vi "2014 Target Detection.vi"() -> (2 "Target Info":T4(array[cluster]))   [LabVIEW 2013]
uses:
  TargetType.ctl
  <vilib>/Rock Robotics/WPI/Camera/WPI_CameraImageSize.ctl
  <vilib>/Rock Robotics/WPI/Camera/WPI_CameraWhite Balance Values.ctl
  <vilib>/Rock Robotics/WPI/Camera/WPI_CameraExposure Values.ctl
  <vilib>/Rock Robotics/WPI/Camera/WPI_CameraFrameRate.ctl
panel:
  in  "Range":cluster{"Lower value":sgl, "Upper value":sgl}={"Lower value"=150.0, "Upper value"=255.0} {"Lower value" scale=0.0..255.0; "Upper value" scale=0.0..255.0}
  in  "Image Size":T1=enum."320x240"
  in  "error in (no error)":errorcluster
  in  "Instructions:":string="Images:\nUse the tab immediately below to choose the image source. Update the camera settings or the image directory so that you have images or video to test with.\n\nCalibration:\nYou can update Color Component ranges directly, or by clicking and drawing a line on the colored strip in the Image control. The Std Dev multipliers and where the strip is drawn determine the calibration values.\n\nUse Debugging tab to view the result of the color range threshold .\n\nArea Size LImit is used to ignore objects too small or far away to care about.\n\nThe Details tab contains score details for each target and subObject.\n\nCamera Type is used to select lens angles for distance calculation.\n\nVertical strips with no adjacent horizontal strip are identified as \"not hot\" and marked in blue.\nThe numeric scores indicate represent aspect ratio and rectangularity.\n\nWhen both strips are near enough, the pair is identified as \"hot\" and marked in green. Scores\nindicate the left, right, ratio of widths, and vertical positioning.\n\nAny score that falls below cutoff is drawn in red and bounding box is drawn in red."
  in  "Std Devs":cluster{"Hue":dbl, "Sat":dbl, "Val":dbl}={"Hue"=4.0, "Sat"=6.0, "Val"=4.0}
  in  "Area Size Limit %":dbl=0.06 format="%#_13g"
  in  "Camera Type":enum16{"206", "1011", "1013"}(ring)=enum."1013"
  out "loop time ms":u32
  in  "Score Cutoff":dbl(slide)=54.248366013071895 scale=0.0..100.0
  in  "Image Source":enum32{"Files", "Camera"}(tab)
  in  "List of image files":i32(listbox)
  in  "Image Directory":path=path "2014 Pseudo-Target/2014 Pseudo-Target Active"
  in  "Tabbed Info":enum32{"Debugging", "Details"}(tab)
  out "Mask":T2(plugin-control)
  out "Image":T2(plugin-control)
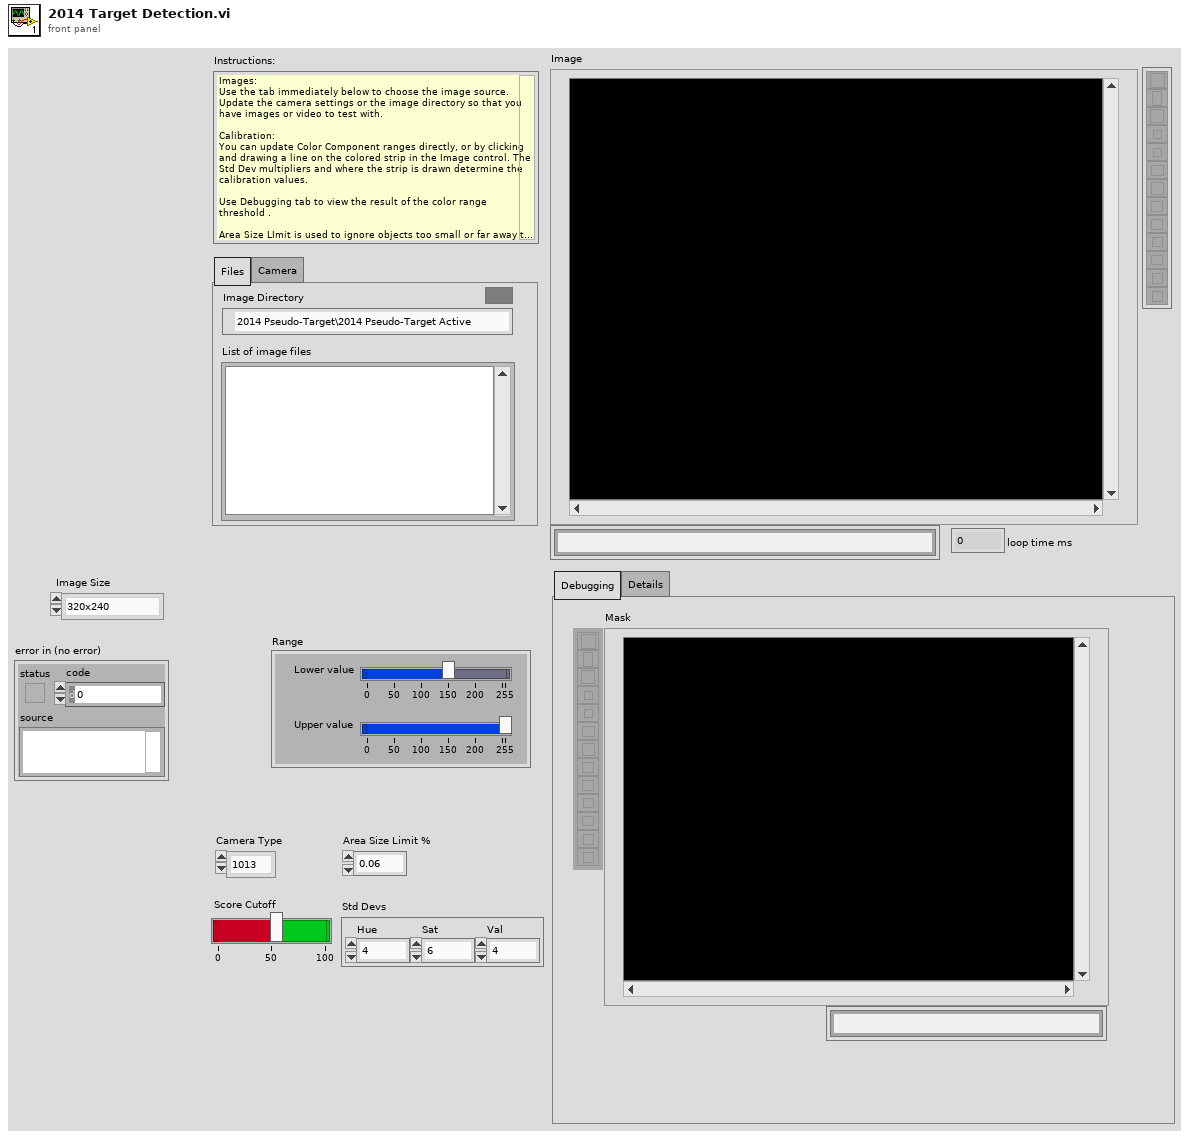
[diagram p1: front panel]
types:
  T1 = typedef "WPI_CameraImageSize.ctl" = enum16{"640x480", "320x240", "160x120"}
  T2 = typedef "IMAQ Image.ctl" = refnum<image>
  T3 = typedef "TargetType.ctl" = enum16{"Not Hot", "Hot"}
  T4 = cluster{"Scores":cluster{"Total":dbl, "Left":dbl, "Right":dbl, "Ratio":dbl, "Vertical":dbl, "index":i32, "State":T3}, "Verticals":cluster{"Horizontal?":bool, "Aspect Score":dbl, "Rect Score":dbl, cluster{"Left":dbl, "Top":dbl, "Right":dbl, "Bottom":dbl}, "Equiv H":dbl, "Equiv V":dbl}, "Horizontals":cluster{"Horizontal?":bool, "Aspect Score":dbl, "Rect Score":dbl, cluster{"Left":dbl, "Top":dbl, "Right":dbl, "Bottom":dbl}, "Equiv H":dbl, "Equiv V":dbl}, "Distance ft":dbl, "Center":cluster{"X":dbl, "Y":dbl}}[]
  T5 = typedef "WPI_CameraFrameRate.ctl" = u32
  T6 = typedef "WPI_CameraExposure Values.ctl" = enum16{"Auto", "Flicker-free 50 Hz", "Flicker-free 60 Hz", "Hold current"}
  T7 = typedef "WPI_CameraWhite Balance Values.ctl" = enum16{"Auto", "Fixed indoor", "Fixed outdoor 1", "Fixed outdoor 2", "Fixed fluorescent 1", "Fixed fluorescent 2", "Hold current"}
  T8 = typedef "Image Type" = u32
  T9 = typedef "WPI_CameraDevRef.ctl" = cluster{"Camera Address":string, "CameraStatus":errorcluster, "Acquire Image Notifier":refnum<notifier>}
  T10 = cluster{"Horizontal":bool, "Aspect Score":dbl, "Rect Score":dbl, cluster{"Left":dbl, "Top":dbl, "Right":dbl, "Bottom":dbl}, "Equiv H":dbl, "Equiv V":dbl}[]
  T11 = cluster{cluster{dbl, dbl}, cluster{dbl, dbl}, cluster{dbl, dbl}}
  T12 = cluster{"Scores":cluster{"Total":dbl, "Left":dbl, "Right":dbl, "Ratio":dbl, "Vertical":dbl, "index":i32, "State":T3}, "Verticals":cluster{"Horizontal?":bool, "Aspect Score":dbl, "Rect Score":dbl, cluster{"Left":dbl, "Top":dbl, "Right":dbl, "Bottom":dbl}, "Equiv H":dbl, "Equiv V":dbl}, "Horizontals":cluster{"Horizontal?":bool, "Aspect Score":dbl, "Rect Score":dbl, cluster{"Left":dbl, "Top":dbl, "Right":dbl, "Bottom":dbl}, "Equiv H":dbl, "Equiv V":dbl}, "Validated":bool}[]
  T13 = cluster{"Scores":cluster{"Total":dbl, "Left":dbl, "Right":dbl, "Ratio":dbl, "Vertical":dbl, "index":i32, "State":T3}, "Verticals":cluster{"Horizontal?":bool, "Aspect Score":dbl, "Rect Score":dbl, cluster{"Left":dbl, "Top":dbl, "Right":dbl, "Bottom":dbl}, "Equiv H":dbl, "Equiv V":dbl}, "Horizontals":cluster{"Horizontal?":bool, "Aspect Score":dbl, "Rect Score":dbl, cluster{"Left":dbl, "Top":dbl, "Right":dbl, "Bottom":dbl}, "Equiv H":dbl, "Equiv V":dbl}, "Distance (ft)":dbl, "Target Center (-1 to 1)":cluster{"X":dbl, "Y":dbl}}[]
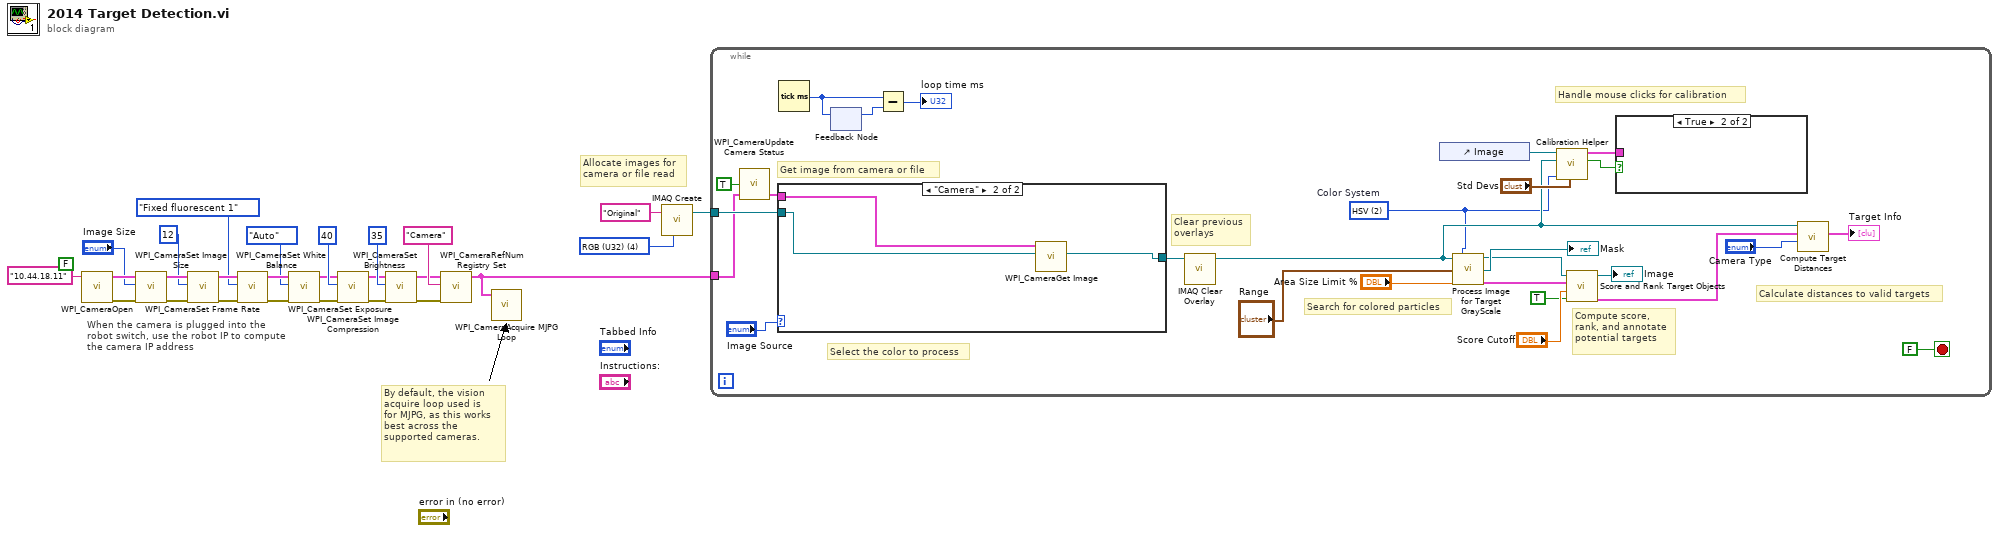
[diagram p0: block diagram]
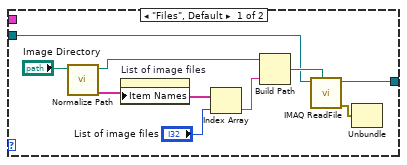
[diagram p3: hidden frame]
diagram:
  (unwired) FALSE ("Disallow Simulation")
  w26 = T8 4 items=["Grayscale (U8)", "Grayscale (I16)", "Grayscale (SGL)", "Complex (CSG)", "RGB (U32)", "HSL (U32)", "RGB (U64)", "Grayscale (U16)"] ("Image Type")
  # "When the camera is plugged into the\nrobot switch, use the robot IP to compute\nthe camera IP address"
  # "By default, the vision\nacquire loop used is\nfor MJPG, as this works\nbest across the\nsupported cameras."
  # "Allocate images for\ncamera or file read"
  n1 = call <vilib>:"WPI_CameraOpen.vi"("Camera Address"="10.44.18.11") -> ("error out"=w14:errorcluster, "CameraDevRef"=w15:T9)  [unwired: 2 in, 7 out]
  n2 = call <vilib>:"WPI_CameraSet Image Size.vi"("error in (no error)"=w14, "Image Size"="Image Size", "CameraDevRef"=w15) -> ("error out"=w13:errorcluster, "CameraDevRef Out"=w16:T9)  [unwired: 7 out]
  n3 = call <vilib>:"WPI_CameraSet Frame Rate.vi"("error in (no error)"=w13, "Frame Rate (fps)"=T5 12, "CameraDevRef"=w16) -> ("error out"=w12:errorcluster, "CameraDevRef Out"=w18:T9)  [unwired: 7 out]
  n4 = call <vilib>:"WPI_CameraSet White Balance.vi"("error in (no error)"=w12, "White Balance"=WPI_CameraWhite_Balance_Values."Fixed fluorescent 1", "CameraDevRef"=w18) -> ("error out"=w11:errorcluster, "CameraDevRef Out"=w17:T9)  [unwired: 7 out]
  n5 = call <vilib>:"WPI_CameraSet Exposure.vi"("error in (no error)"=w11, "Exposure"=WPI_CameraExposure_Values."Auto", "CameraDevRef"=w17) -> ("error out"=w10:errorcluster, "CameraDevRef Out"=w20:T9)  [unwired: 7 out]
  n6 = call <vilib>:"WPI_CameraSet Image Compression.vi"("error in (no error)"=w10, "Compression"=40, "CameraDevRef"=w20) -> ("error out"=w9:errorcluster, "CameraDevRef Out"=w19:T9)  [unwired: 7 out]
  n7 = call <vilib>:"WPI_CameraSet Brightness.vi"("error in (no error)"=w9, "Brightness"=35, "CameraDevRef"=w19) -> ("error out"=w7:errorcluster, "CameraDevRef Out"=w8:T9)  [unwired: 7 out]
  n8 = call <vilib>:"WPI_CameraRefNum Registry Set.vi"("error in (no error)"=w7, "refnum name"="Camera", "CameraDevRef"=w8) -> ("CameraDevRef"=w2:T9)  [unwired: 8 out]
  n9 = call <vilib>:"WPI_CameraAcquire MJPG Loop.vi"("CameraDevRef"=w2) -> ()  [unwired: 11 in]
  n10 = call "IMAQ Create"("Image Name"="Original", "Image Type"=w26) -> ("New Image"=w24:T2)  [unwired: 3 in, 1 out]
  n11 = while {
    tunnel: w24 -> [w50]
    tunnel: w2 -> [w36]
    stop <- FALSE stop-if-true
    w29 = u16 2 items=["RGB", "HSL", "HSV", "HSI"]  # Color System
    # "Clear previous\noverlays"
    # "Calculate distances to valid targets"
    # "Search for colored particles"
    # "Handle mouse clicks for calibration"
    # "Compute score,\nrank, and annotate\npotential targets"
    # "Select the color to process"
    # "Get image from camera or file"
    n12 = call <vilib>:"WPI_CameraUpdate Camera Status.vi"("CameraDevRef In"=w36, "Enable Vision"=TRUE) -> ("CameraDevRef Out"=w34:T9)  [unwired: 3 in]
    n13 = case shown="\"Camera\"" "Image Source" {
      tunnel: [w59 w65] -> w53
      tunnel: w50 -> [w58 w63]
      tunnel: w34 -> [_ w64]
      frame "Files", Default {
        n14 = call "Normalize Path.vi"("Image Directory"="Image Directory") -> ("Filenames"=w55:string[], "Path"=w54:path)  [unwired: 9 in]
        n15 = property on="List of image files" class="LstBox (strict)"("Item Names"=w55) -> ()  [unwired: 2 in, 2 out]
        n16 = Index Array(array=w55, index="List of image files") -> (element=w61:string)
        n17 = Build Path(base path=w54, name or relative path=w61) -> (appended path=w60:path)
        n18 = call "IMAQ ReadFile"("File Path"=w60, "Image"=w58) -> ("error out"=w57:errorcluster, "Image Out"=w59:T2)  [unwired: 5 in, 3 out]
        n19 = Unbundle(w57) -> ()  [unwired: 3 out]
      }
      frame "Camera" {
        n20 = call <vilib>:"WPI_CameraGet Image.vi"("Image"=w63, "CameraDevRef"=w64) -> ("Image Out"=w65:T2)  [unwired: 1 in, 8 out]
      }
    }
    n21 = Tick Count (ms)() -> (millisecond timer value=w49:u32)
    n22 = feedback #1() -> (w48:u32)  [unwired: 1 in]
    n23 = feedback-in #1(w49) -> ()
    n24 = Subtract(x=w49, y=w48) -> (x-y=→"loop time ms":u32)
    n25 = call "IMAQ Clear Overlay"("Image"=w53) -> ("Image Out"=w33:T2)  [unwired: 9 in, 1 out]
    n26 = control-ref of="Image"() -> (w41:refnum<vi>)
    n27 = call "Process Image for Target GrayScale.vi"("Src Image"=w33, "Color Mode"=w29, "Range"="Range", "Area Cutoff %"="Area Size Limit %") -> ("Src Image Out"=w31:T2, "Threshold"=→"Mask":T2, "Particles"=w30:T10)  [unwired: 9 in]
    n28 = call "Calibration Helper.vi"("Std Devs"="Std Devs", "Color Mode"=w29, "Image"=w33, "Image Ctl Refnum"=w41) -> ("Changed"=w38:bool, "output color"=w39:T11)  [unwired: 6 in]
    n29 = call "Score and Rank Target Objects.vi"("Annotate"=TRUE, "Score Limit"="Score Cutoff", "Particles"=w30, "Image in"=w31) -> ("Target Info"=w44:T12, "Annotated Image"=→"Image":T2)  [unwired: 6 in]
    n30 = case shown="True" w38 {
      tunnel: w39 -> [_ _]
      frame False {
      }
      frame True {
      }
    }
    n31 = call "Compute Target Distances.vi"("Camera Type"="Camera Type", "Target Info"=w44, "Image in"=w33) -> ("Target Info"=→"Target Info":T13)  [unwired: 6 in, 2 out]
  }
